vi "get RW State.vi"(11 "IO in":refnum<class "IO.lvclass">) -> (3 "R/W State":bool)   [LabVIEW 2021, in "IO.lvclass"]
uses:
  IO.lvclass
  IO.lvclass/IO.ctl
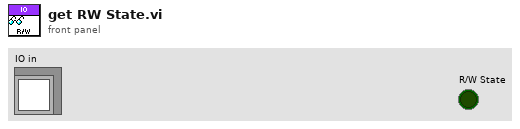
[diagram p1: front panel]
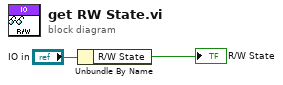
[diagram p0: block diagram]
diagram:
  n1 = Unbundle By Name("IO in") -> ("R/W State"=→"R/W State":bool)
